vi "WLC fitting_twoside_YCC.vi"(4 "QPD-y":dbl[](array[numeric]), 5 "QPD-x":dbl[](array[numeric]), 6 "Xstage":dbl[](array[numeric]), 7 "T=Read data mode?\nF=Real time fit":bool=TRUE) -> ()   [LabVIEW 2014]
doc: "This VI utilizes the LabVIEW implemented non-linear curve fitting algorithm to fit worm-like chain model. \nThere are 2 modes can be selected: one is real-time fitting mode, the other is data reading mode. \n\nIn the real-time fitting mode, the force-extension assay VI will automatically pass the data and the settings into this VI, and then fitting. \n\nIn the data reading mode, you should first select the data path to read, and manually input all the setting, such as height and fitting range, and then push the \"run\" button. \n\nThe VI will calculate the DNA extension, and extract the pre-set fitting range to do WLC fitting. The data output includes contour length, persistence length, fitted center, recorded data and fitted data."
uses:
  <vilib>/gmath/NI_Gmath.lvlib
  <vilib>/Utility/file.llb/Read From Spreadsheet File (DBL).vi
  <vilib>/Utility/file.llb/Write To Spreadsheet File (DBL).vi
  <vilib>/gmath/NumericalOptimization/Nonlinear Curve Fit LM formula string.vi
  SubVI/WLC-Fitting Cluster.ctl
panel:
  out "output cluster":T1={"cr (um)"=0.0, "yr (V)"=0.0, "trap height(nm)"=0.0, "bead radius(nm)"=520.0, "Length offset"=0.0, "Force offset"=0.0, "cr shift (nm)"=0.0, "yr shift (mV)"=0.0, "LaserPower (mW)"=0.0, "conversion factor (V/um)"=0.0, "Stiffness (pN/nm)"=0.0154}
  in  "stuckbead path (dialog if empty)":path
  in  "Fitting Cluster":T2={"cr (um)"=0.0, "yr (V)"=0.0, "trap height(nm)"=300.0, "bead radius(nm)"=515.0, "Length offset"=400.0, "conversion factor (V/um)"=0.0, "Force constant (pN/nm)"=0.0154, "Force offset"=10.0, "cr shift (nm)"=0.0, "yr shift (mV)"=0.0, "LaserPower (mW)"=40.0, "Cf. Calib. Array"=[], "Stiffness Calib. array"=[0.0032, 0.00095]}
  out "Tether QPD height":dbl
  in  "initial parameters for fit K":dbl[](array[numeric])=[40.0, 1150.0]
  in  "initial parameters 2":dbl[](array[numeric])=[40.0, 1150.0]
  in  "Enum":T3(ring)
  out "residue":dbl
  in  "Tab Control 2":enum32{"Page 1"}(tab)
  in  "T=positive (RHS)\nF=negative (LHS)":bool
  in  "fit only one side?":bool
  in  "OK to fit?":bool
  in  "X=T,Y=F":bool=TRUE
  in  "Tab Control":T4(tab)
  out "Stuckbead Scan":cluster{"all rows":dbl[], "all rows":dbl[]}(graph)
  out "Rbead vs zbd":cluster{"all rows":dbl[], "all rows":dbl[]}(graph)
  out "XY Graph 2":T5(graph)
  out "XY Graph":cluster{"Y":dbl[], "Y":dbl[]}[](graph)
  out "XY Graph 3":cluster{"xDNA-cut":dbl[], "Force-cut":dbl[]}[](graph)
  in  "stop to save?":bool
  in  "initial parameters for marko":dbl[](array[numeric])=[40.0, 1150.0, 0.001, 0.001]
  out "yi":dbl
  out "Position Array Out":dbl[](array[numeric])
  in  "F-x data":path
  out "ci":dbl
  in  "Save fit?":bool
  out "QPD signal Out":dbl[](array[numeric])
  out "position-QPD":T6(graph)
  out "best fit parameters":dbl[](array[numeric])
  # "1750.8 nm for 5180 bp\n1109.0 nm for 3281bp"
  # "Lp"
  # "L0"
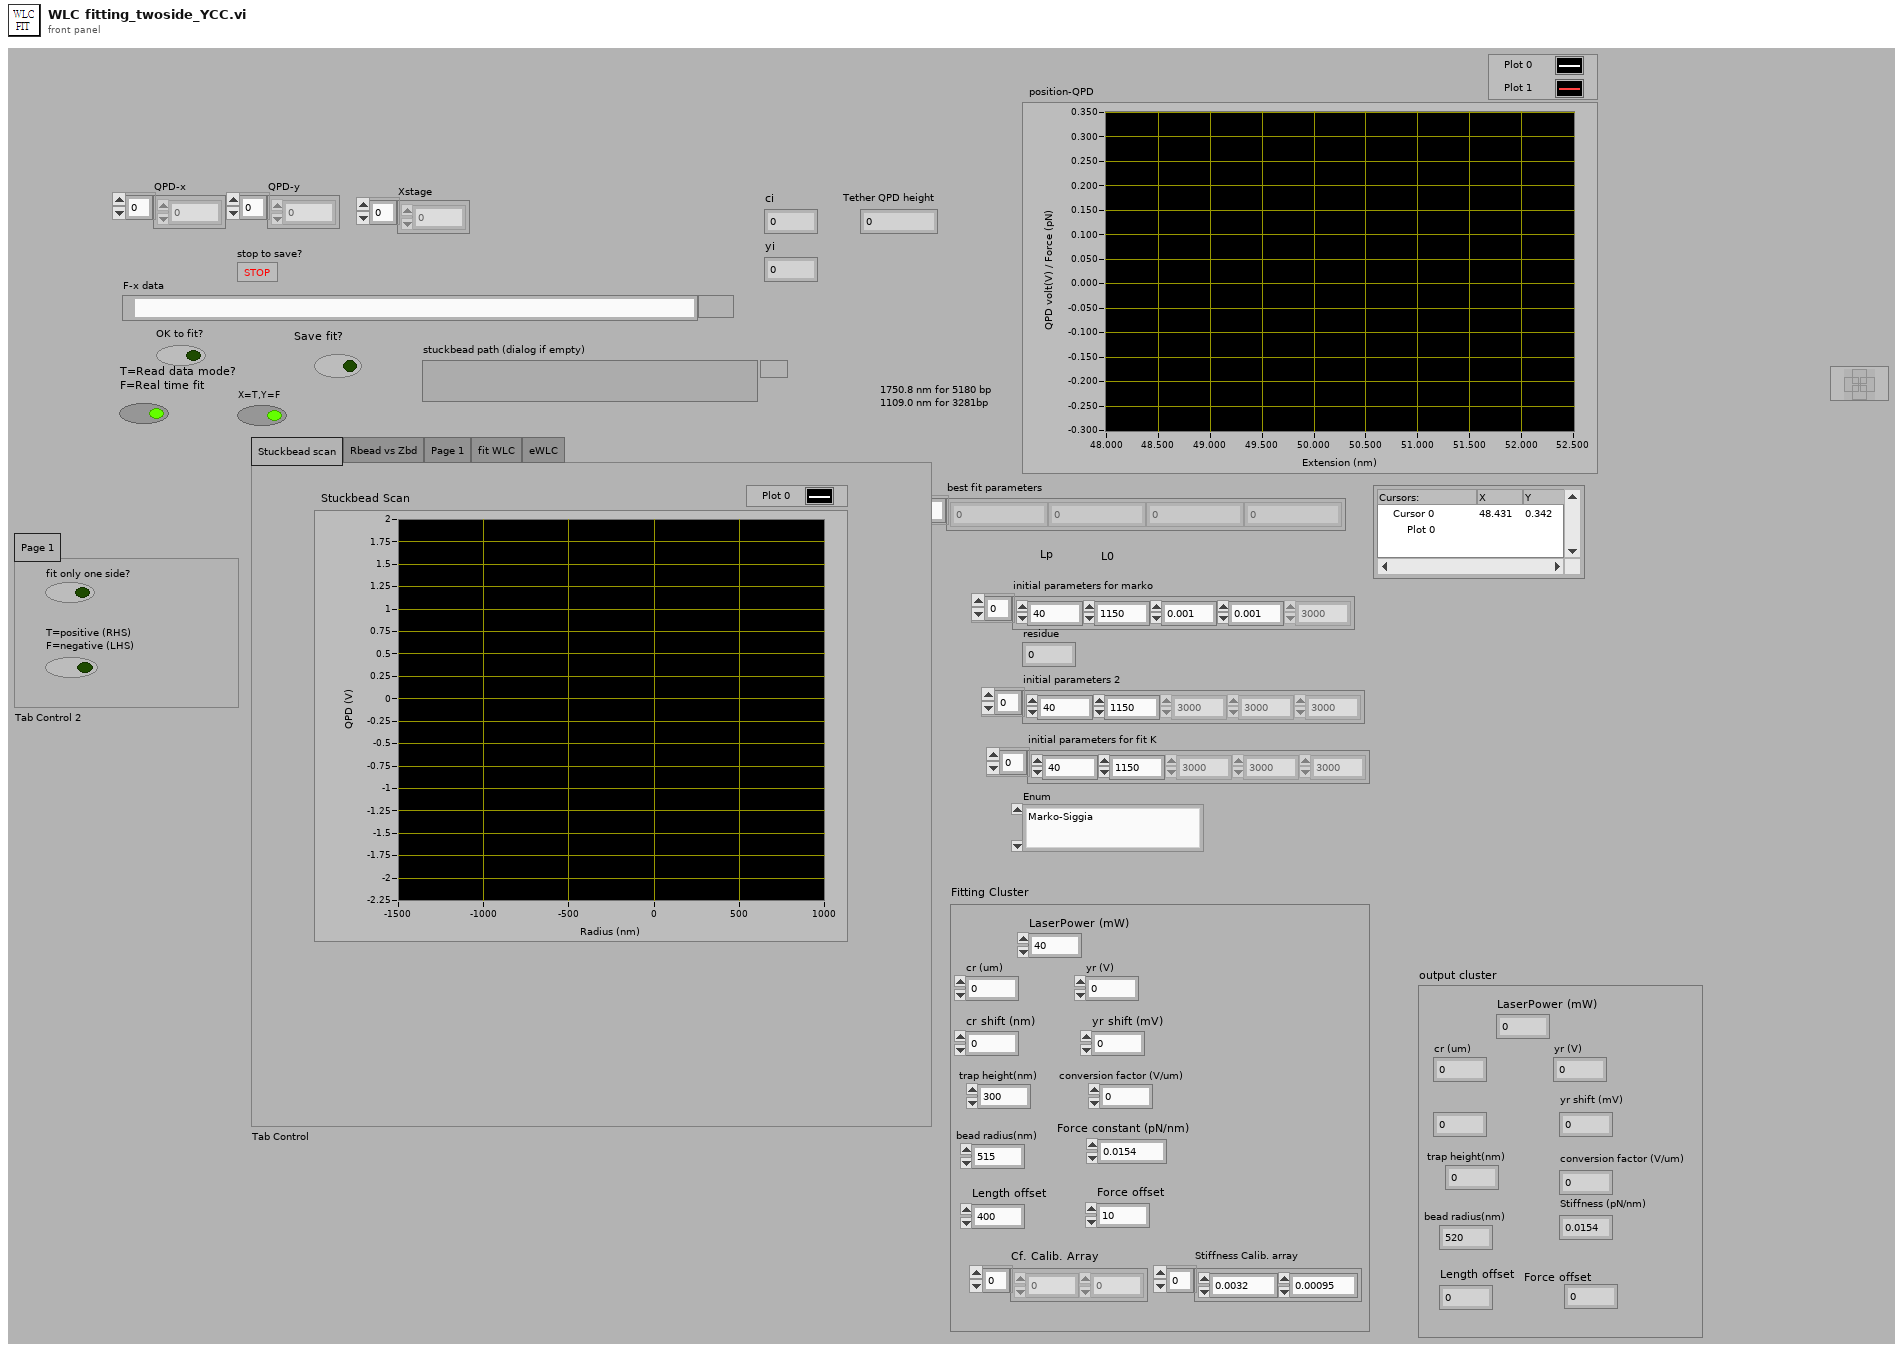
[diagram p1: front panel]
types:
  T1 = typedef "WLC-Fitting Cluster.ctl" = cluster{"cr (um)":dbl, "yr (V)":dbl, "trap height(nm)":dbl, "bead radius(nm)":dbl, "Length offset":dbl, "Force offset":dbl, "cr shift (nm)":dbl, "yr shift (mV)":dbl, "LaserPower (mW)":dbl, "conversion factor (V/um)":dbl, "Stiffness (pN/nm)":dbl}
  T2 = typedef "WLC-Fitting Cluster.ctl" = cluster{"cr (um)":dbl, "yr (V)":dbl, "trap height(nm)":dbl, "bead radius(nm)":dbl, "Length offset":dbl, "conversion factor (V/um)":dbl, "Force constant (pN/nm)":dbl, "Force offset":dbl, "cr shift (nm)":dbl, "yr shift (mV)":dbl, "LaserPower (mW)":dbl, "Cf. Calib. Array":dbl[], "Stiffness Calib. array":dbl[]}
  T3 = enum16{"Marko-Siggia", "modified Marko", "eWLC", "eWLC-modified M-S", "K fit eWLC-modified M-S"}
  T4 = enum32{"Stuckbead scan", "Rbead vs Zbd", "Page 1", "fit WLC", "eWLC"}
  T5 = cluster{"cut-full xDNA":dbl[], "cut-full Force":dbl[]}
  T6 = cluster{"QPD signal Out":dbl[], "Position Array Out":dbl[]}
  T7 = cluster{"Position Array Out":dbl[], "QPD signal Out":dbl[]}
  T8 = cluster{"model":string, "Parameters":string[], "x":string}
  T9 = cluster{"Bead radius (nm)":dbl[], "all rows":dbl[]}
  T10 = cluster{"xDNA-cut":dbl[], "best nonlinear fit":dbl[]}
  T11 = cluster{"best nonlinear fit":dbl[], "Force-cut":dbl[]}
  T12 = cluster{"xDNA-cut":dbl[], "best nonlinear fit":dbl[]}[]
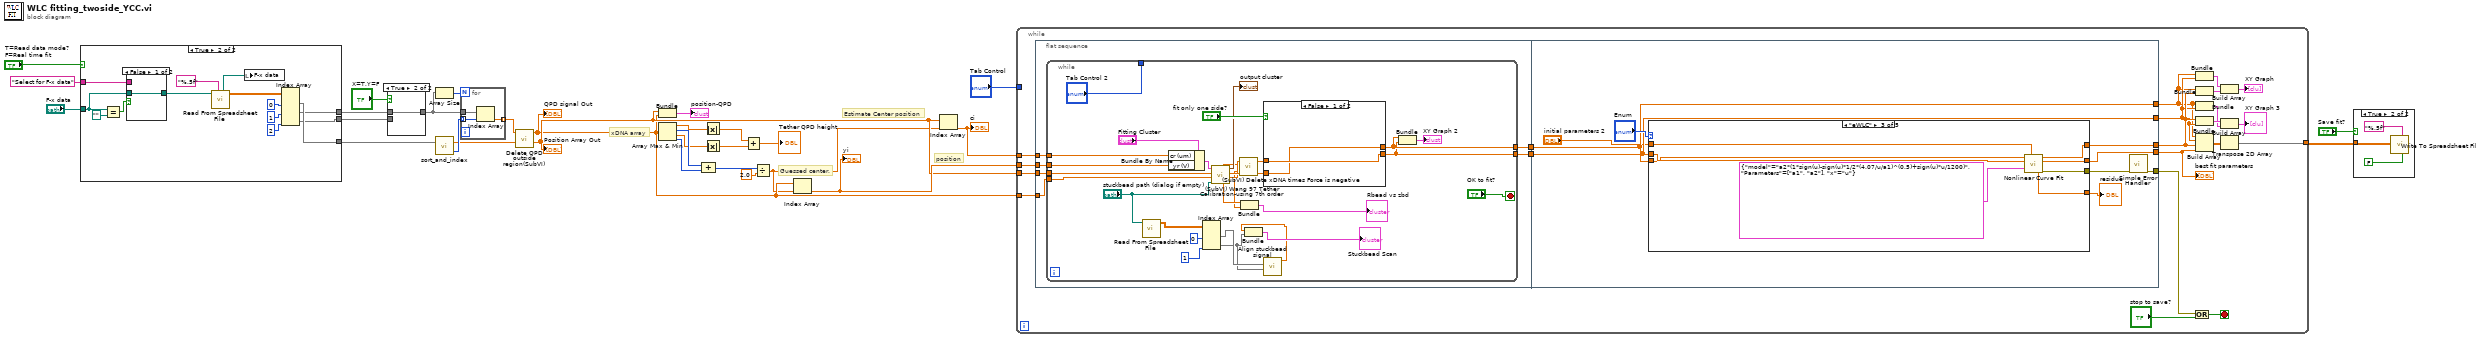
[diagram p0: block diagram]
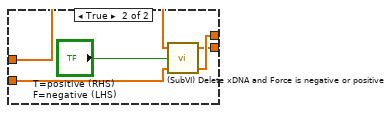
[diagram p2: hidden frame]
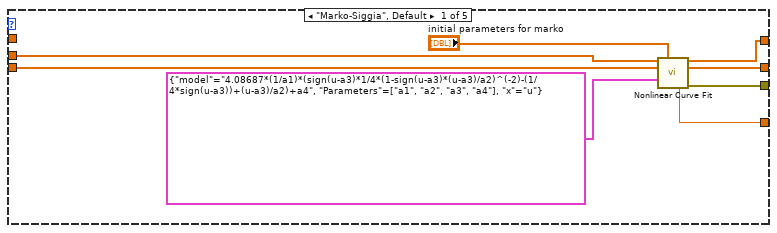
[diagram p3: hidden frame]
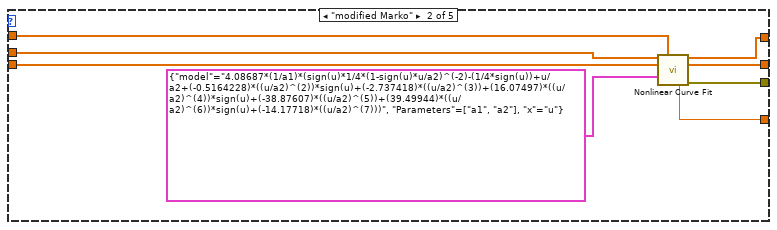
[diagram p4: hidden frame]
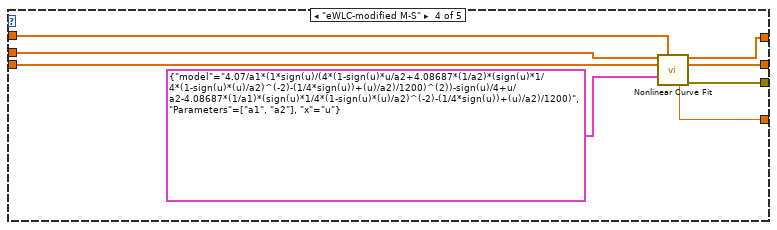
[diagram p5: hidden frame]
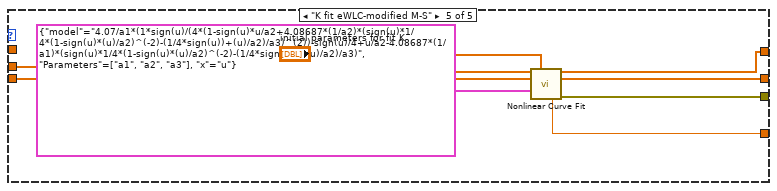
[diagram p6: hidden frame]
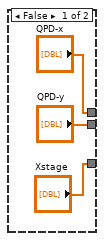
[diagram p8: hidden frame]
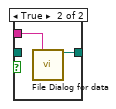
[diagram p9: hidden frame]
diagram:
  # "xDNA array"
  # "Guessed center."
  # "Estimate Center position"
  # "position"
  n1 = case shown="True" "T=Read data mode?\nF=Real time fit" {
    tunnel: ["QPD-x" w41] -> w27
    tunnel: ["QPD-y" w42] -> w26
    tunnel: ["Xstage" w43] -> w18
    tunnel: "Select for F-x data" ("default name") -> [_ w38]
    tunnel: "F-x data" -> [_ w35]
    frame False {
    }
    frame True {
      n2 = Equal?(x=w35, y=path "") -> (x = y?=w36:bool)
      n3 = case shown="False" w36 {
        tunnel: [w48 w49] -> w39
        tunnel: w38 -> [_ w50]
        tunnel: w35 -> [w48 _]
        frame False {
        }
        frame True {
          n4 = call "File Dialog for data"("prompt"=w50) -> ("selected path"=w49:path)  [unwired: 11 in, 3 out]
        }
      }
      n5 = call-poly <vilib>:"Read From Spreadsheet File.vi"("format (%.3f)"="%.5f", "file path (dialog if empty)"=w39) -> ("all rows"=w47:dbl[][], "new file path (Not A Path if cancelled)"=w34:path)  [unwired: 5 in, 3 out]
      n6 = local write "F-x data"(w34) -> ()
      n7 = Index Array(array=w47, index (col) #1=0 ("disabled index (col)"), index (col) #2=1 ("index (col)"), index (col) #3=2 ("index (col)")) -> (element #1=w43:dbl[], element #2=w41:dbl[], element #3=w42:dbl[])  [unwired: 3 in]
    }
  }
  n8 = case shown="True" "X=T,Y=F" {
    tunnel: w26 -> [w51 _]
    tunnel: [w51 w52] -> w15
    tunnel: w27 -> [_ w52]
    frame False {
    }
    frame True {
    }
  }
  n9 = Array Size(array=w15) -> (size(s)=w14:i32)
  n10 = call "sort_and_index.vi"("Presorted Array"=w18) -> ("Index"=w17:i32[], "Sorted Array"=w16:dbl[])  [unwired: 1 in]
  n11 = for {
    N: w14 -> [_]
    tunnel: w15 -> [w55]
    tunnel: w17 -> [w54] mode=indexing
    tunnel: [w53] -> w13 mode=indexing
    n12 = Index Array(array=w55, index=w54) -> (element=w53:dbl)
  }
  n13 = call "Delete QPD outside region(SubVI).vi"("Position Array In"=w16, "QPD signal In"=w13) -> ("Position Array Out"=w12:dbl[], "QPD signal Out"=w11:dbl[])  [unwired: 8 in]
  "QPD signal Out" <- w11
  "Position Array Out" <- w12
  n14 = Bundle("Position Array Out"=w12, "QPD signal Out"=w11) -> (→"position-QPD":T7)  [unwired: 1 in]
  n15 = Array Max & Min(array=w11) -> (max value=w5:dbl, max index (indices)=w10:i32, min value=w4:dbl, min index (indices)=w9:i32)
  n16 = Compound Arithmetic op=ADD(w10, w9) -> (w30:i32)
  n17 = Absolute Value(x=w5) -> (abs(x)=w3:dbl)
  n18 = Absolute Value(x=w4) -> (abs(x)=w2:dbl)
  n19 = Add(x=w3, y=w2) -> (x+y=→"Tether QPD height":dbl)
  n20 = Divide(x=w30, y=2.0) -> (x/y=w8:dbl)
  n21 = Index Array(array=w11, index=w8) -> (element=w20:dbl)
  "yi" <- w20
  n22 = Index Array(array=w12, index=w8) -> (element=w21:dbl)
  "ci" <- w21
  n23 = while {
    tunnel: [w75] -> w23
    tunnel: w12 -> [w73]
    tunnel: w11 -> [w71]
    tunnel: w21 -> [w70]
    tunnel: w20 -> [w69]
    tunnel: "Tab Control" -> [_]
    stop <- w67 stop-if-true
    n24 = flat-sequence {
      tunnel: w73 -> [w82]
      tunnel: w71 -> [w81]
      tunnel: w70 -> [w80]
      tunnel: w69 -> [w79]
      tunnel: [w78] -> w66
      tunnel: [w77] -> w65
      tunnel: [w125] -> w58
      tunnel: w66 -> [w123]
      tunnel: w65 -> [w125]
      tunnel: [w124] -> w61
      tunnel: [w123] -> w59
      tunnel: [w122] -> w64
      tunnel: [w120] -> w63
      frame #0 {
        n25 = while {
          tunnel: w82 -> [w102]
          tunnel: w81 -> [w103]
          tunnel: w80 -> [w99]
          tunnel: w79 -> [w98]
          tunnel: [w105] -> w78
          tunnel: [w106] -> w77
          tunnel: ["Tab Control 2"] -> _
          stop <- "OK to fit?" stop-if-true
          n26 = call-poly <vilib>:"Read From Spreadsheet File.vi"("file path (dialog if empty)"="stuckbead path (dialog if empty)") -> ("all rows"=w92:dbl[][])  [unwired: 6 in, 4 out]
          n27 = Bundle By Name(cluster="Fitting Cluster", "cr (um)"=w99, "yr (V)"=w98) -> (w97:T2)
          n28 = Index Array(array=w92, index (col) #1=0 ("disabled index (col)"), index (col) #2=1 ("disabled index (col)")) -> (element #1=w85:dbl[], element #2=w84:dbl[])  [unwired: 2 in]
          n29 = call "(SubVI) Wang 97 Tether Calibration-using 7th order.vi"("stuckbead path (dialog if empty)"="stuckbead path (dialog if empty)", "QPD signal"=w103, "Stage Position"=w102, "Fitting Cluster"=w97) -> ("Force"=w95:dbl[], "xDNA"=w96:dbl[], "output cluster"=→"output cluster":T1, "Xbead (nm)"=w88:dbl[], "zbd (nm)"=w87:dbl[])  [unwired: 3 in]
          n30 = call "(SubVI) Delete xDNA times Force is negative.vi"("xDNA"=w96, "Force"=w95) -> ("xDNA-cut"=w107:dbl[], "Force-cut"=w108:dbl[])  [unwired: 2 in]
          n31 = Bundle("Xbead (nm)"=w88, "zbd (nm)"=w87) -> (→"Rbead vs zbd":cluster{"Xbead (nm)":dbl[], "zbd (nm)":dbl[]})  [unwired: 1 in]
          n32 = call "Align stuckbead signal.vi"("stuckbstuck QPD (V)"=w84, "Stage (um)"=w85) -> ("Bead radius (nm)"=w83:dbl[])  [unwired: 3 in, 1 out]
          n33 = Bundle("Bead radius (nm)"=w83, "all rows"=w84) -> (→"Stuckbead Scan":T9)  [unwired: 1 in]
          n34 = case shown="False" "fit only one side?" {
            tunnel: w108 -> [w112 w117]
            tunnel: w107 -> [w111 w115]
            tunnel: [w111 w114] -> w106
            tunnel: [w112 w113] -> w105
            frame False {
            }
            frame True {
              n35 = call "(SubVI) Delete xDNA and Force is negative or positive.vi"("xDNA"=w115, "T=positive (RHS)\nF=negative (LHS)"="T=positive (RHS)\nF=negative (LHS)", "Force"=w117) -> ("xDNA-cut"=w114:dbl[], "Force-cut"=w113:dbl[])  [unwired: 1 in]
            }
          }
          n36 = Bundle("xDNA-cut"=w106, "Force-cut"=w105) -> (→"XY Graph 2":cluster{"xDNA-cut":dbl[], "Force-cut":dbl[]})  [unwired: 1 out]
        }
      }
      frame #1 {
        n37 = case shown="\"eWLC\"" "Enum" {
          tunnel: "initial parameters 2" -> [_ w141 w147 w157 _]
          tunnel: w123 -> [w133 w139 w149 w155 w165]
          tunnel: w125 -> [w132 w140 w148 w156 w164]
          tunnel: [w131 w136 w145 w151 w159] -> w124
          tunnel: [w130 w137 w146 w152 w160] -> w122
          tunnel: [w129 w138 w144 w153 w161] -> w121
          tunnel: [w128 w135 w143 w154 w162] -> w119
          frame "Marko-Siggia", Default {
            n38 = call-poly <vilib>:"Nonlinear Curve Fit.vi"("Y"=w133, "initial parameters"="initial parameters for marko", "X"=w132, "model description"=T8 {"model"="4.08687*(1/a1)*(sign(u-a3)*1/4*(1-sign(u-a3)*(u-a3)/a2)^(-2)-(1/4*sign(u-a3))+(u-a3)/a2)+a4", "Parameters"=["a1", "a2", "a3", "a4"], "x"="u"}) -> ("best nonlinear fit"=w131:dbl[], "best fit parameters"=w130:dbl[], "residue"=w128:dbl, "error out"=w129:errorcluster)  [unwired: 3 in, 5 out]
          }
          frame "modified Marko" {
            n39 = call-poly <vilib>:"Nonlinear Curve Fit.vi"("Y"=w139, "initial parameters"=w141, "X"=w140, "model description"=T8 {"model"="4.08687*(1/a1)*(sign(u)*1/4*(1-sign(u)*u/a2)^(-2)-(1/4*sign(u))+u/a2+(-0.5164228)*((u/a2)^(2))*sign(u)+(-2.737418)*((u/a2)^(3))+(16.07497)*((u/a2)^(4))*sign(u)+(-38.87607)*((u/a2)^(5))+(39.49944)*((u/a2)^(6))*sign(u)+(-14.17718)*((u/a2)^(7)))", "Parameters"=["a1", "a2"], "x"="u"}) -> ("best nonlinear fit"=w136:dbl[], "best fit parameters"=w137:dbl[], "residue"=w135:dbl, "error out"=w138:errorcluster)  [unwired: 3 in, 5 out]
          }
          frame "eWLC" {
            n40 = call-poly <vilib>:"Nonlinear Curve Fit.vi"("Y"=w148, "initial parameters"=w147, "X"=w149, "model description"=T8 {"model"="a2*(1*sign(u)-sign(u)*1/2*(4.07/u/a1)^(0.5)+sign(u)*u/1200)", "Parameters"=["a1", "a2"], "x"="u"}) -> ("best nonlinear fit"=w145:dbl[], "best fit parameters"=w146:dbl[], "residue"=w143:dbl, "error out"=w144:errorcluster)  [unwired: 3 in, 5 out]
          }
          frame "eWLC-modified M-S" {
            n41 = call-poly <vilib>:"Nonlinear Curve Fit.vi"("Y"=w155, "initial parameters"=w157, "X"=w156, "model description"=T8 {"model"="4.07/a1*(1*sign(u)/(4*(1-sign(u)*u/a2+4.08687*(1/a2)*(sign(u)*1/4*(1-sign(u)*(u)/a2)^(-2)-(1/4*sign(u))+(u)/a2)/1200)^(2))-sign(u)/4+u/a2-4.08687*(1/a1)*(sign(u)*1/4*(1-sign(u)*(u)/a2)^(-2)-(1/4*sign(u))+(u)/a2)/1200)", "Parameters"=["a1", "a2"], "x"="u"}) -> ("best nonlinear fit"=w151:dbl[], "best fit parameters"=w152:dbl[], "residue"=w154:dbl, "error out"=w153:errorcluster)  [unwired: 7 in, 1 out]
          }
          frame "K fit eWLC-modified M-S" {
            n42 = call-poly <vilib>:"Nonlinear Curve Fit.vi"("Y"=w165, "initial parameters"="initial parameters for fit K", "X"=w164, "model description"=T8 {"model"="4.07/a1*(1*sign(u)/(4*(1-sign(u)*u/a2+4.08687*(1/a2)*(sign(u)*1/4*(1-sign(u)*(u)/a2)^(-2)-(1/4*sign(u))+(u)/a2)/a3)^(2))-sign(u)/4+u/a2-4.08687*(1/a1)*(sign(u)*1/4*(1-sign(u)*(u)/a2)^(-2)-(1/4*sign(u))+(u)/a2)/a3)", "Parameters"=["a1", "a2", "a3"], "x"="u"}) -> ("best nonlinear fit"=w159:dbl[], "best fit parameters"=w160:dbl[], "residue"=w162:dbl, "error out"=w161:errorcluster)  [unwired: 7 in, 1 out]
          }
        }
        "residue" <- w119
        n43 = call <vilib>:"Simple Error Handler.vi"("error in (no error)"=w121) -> ("error out"=w120:errorcluster)  [unwired: 4 in, 4 out]
      }
    }
    n44 = Or(x=w63, y="stop to save?") -> (x .or. y?=w67:bool)
    n45 = Bundle("xDNA-cut"=w58, "Force-cut"=w59) -> (w74:cluster{"xDNA-cut":dbl[], "Force-cut":dbl[]})  [unwired: 1 out]
    n46 = Bundle("xDNA-cut"=w58, "best nonlinear fit"=w61) -> (w72:T10)  [unwired: 1 out]
    n47 = Bundle("xDNA-cut"=w58, "Force-cut"=w59) -> (w57:cluster{"xDNA-cut":dbl[], "Force-cut":dbl[]})  [unwired: 1 out]
    n48 = Bundle("best nonlinear fit"=w61, "Force-cut"=w59) -> (w60:T11)  [unwired: 1 out]
    n49 = Build Array(w58, w59, w61, w64) -> (w76:dbl[][])
    n50 = Build Array(w74, w72) -> (→"XY Graph":T12)
    n51 = Build Array(w60, w57) -> (→"XY Graph 3":cluster{"xDNA-cut":dbl[], "Force-cut":dbl[]}[])
    n52 = Transpose 2D Array(2D array=w76) -> (transposed array=w75:dbl[][])
    "best fit parameters" <- w64
  }
  n53 = case shown="True" "Save fit?" {
    tunnel: w23 -> [_ w167]
    frame False {
    }
    frame True {
      n54 = call-poly <vilib>:"Write To Spreadsheet File.vi"("transpose? (no:F)"=FALSE, "format (%.3f)"="%.5f", "2D data"=w167) -> ()  [unwired: 5 in, 1 out]
    }
  }
